vi "Initialize DO.vi"(0 "DAQ":refnum<class "DAQ.lvclass">, 5 "DAQNode Dict":T1, 7 "DO Channels":T2[](array[typedef]), 11 "error in":errorcluster, 14 "Simulate":bool) -> (4 "DAQ out":refnum<class "DAQ.lvclass">, 6 "DAQNode Dict out":T1, 15 "error out":errorcluster)   [LabVIEW 2017, in "DAQ.lvclass"]
doc: "Developed by Kevin Thompson\nkevin@thompsonengineering.net\n\nCopyright 2015\nThompson Engineering, LLC"
uses:
  DAQ.lvclass
  DataTypes/TD DO Channel--cluster.ctl
  <vilib>/TELLC/Dynamic CVT API/TD Dynamic CVT DVR--ref.ctl
  DAQ.lvclass/DAQ.ctl
  Accessors/Set DO IONames.vi
  Accessors/Set DO SchemNames.vi
  <vilib>/DAQmx/create/channels.llb/DAQmx Create Channel (DO-Digital Output).vi
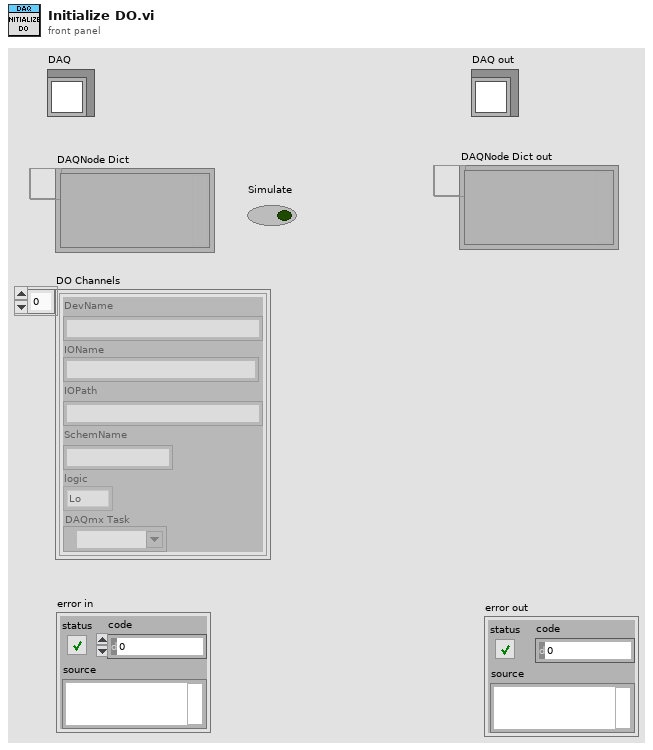
[diagram p1: front panel]
types:
  T1 = typedef "TD Dynamic CVT DVR--ref.ctl" = refnum<data-value>
  T2 = typedef "DAQ.lvclass/TD DO Channel--cluster.ctl" = cluster{"DevName":string, "IOName":string, "IOPath":string, "SchemName":string, "logic":enum16{"Lo", "Hi"}, "DAQmx Task":refnum<k21>}
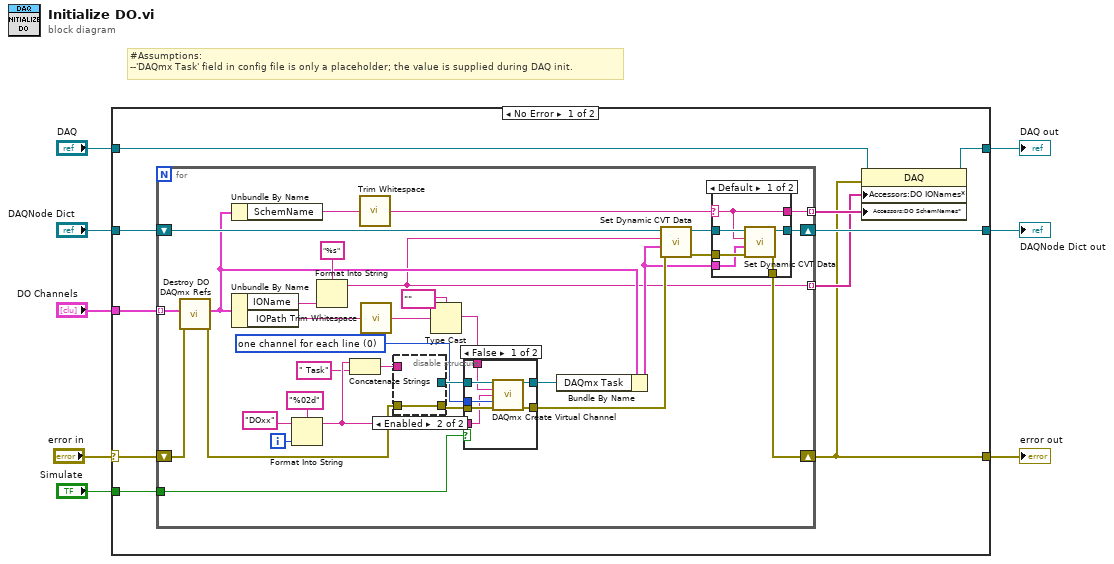
[diagram p0: block diagram]
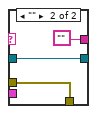
[diagram p2: hidden frame]
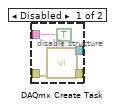
[diagram p3: hidden frame]
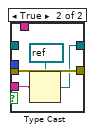
[diagram p4: hidden frame]
diagram:
  # "#Assumptions:\n--'DAQmx Task' field in config file is only a placeholder; the value is supplied during DAQ init."
  n1 = case shown="No Error" "error in" {
    selector: "error in" -> [w17 w79]
    tunnel: "DO Channels" -> [w16 _]
    tunnel: "DAQNode Dict" -> [w18 w78]
    tunnel: [w12 w79] -> w6
    tunnel: [w15 w78] -> w5
    tunnel: "Simulate" -> [w9 _]
    tunnel: "DAQ" -> [w11 w77]
    tunnel: [w10 w77] -> w1
    frame No Error {
      n2 = for {
        tunnel: w16 -> [w36] mode=indexing
        shift-right: [w26] -> w12
        shift-left: w17 -> [w35]
        shift-right: [w28] -> w15
        shift-left: w18 -> [w44]
        tunnel: [w21] -> w14 mode=indexing
        tunnel: [w20] -> w13 mode=indexing
        tunnel: w9 -> [w19]
        i -> [w47]
        w42 = 0 items=["one channel for each line", "one channel for all lines"] ("line grouping")
        n3 = call "Destroy DO DAQmx Refs.vi"("error in (no error)"=w35, "DO"=w36) -> ("error out"=w34:errorcluster, "DO out"=w24:T2)  [unwired: 8 in]
        n4 = Unbundle By Name(w24) -> ("SchemName"=w23:string)
        n5 = Unbundle By Name(w24) -> ("IOName"=w33:string, "IOPath"=w49:string)
        n6 = Format Into String(format string="%02d", initial string="DOxx", w47) -> (resulting string=w39:string)  [unwired: 1 in, 1 out]
        n7 = Format Into String(format string="%s", w33) -> (resulting string=w20:string)  [unwired: 2 in, 1 out]
        n8 = Concatenate Strings(w39, " Task" ("string")) -> (w37:string)
        n9 = call <vilib>:"Trim Whitespace.vi"("string"=w23) -> ("trimmed string"=w22:string)  [unwired: 1 in]
        n10 = call <vilib>:"Trim Whitespace.vi"("string"=w49) -> ("trimmed string"=w48:string)  [unwired: 1 in]
        n11 = disable-structure shown="Enabled" {
          disable-tunnel: [w64 _] -> w50
          disable-tunnel: [w63 w65] -> w45
          disable-tunnel: w37 -> [w62 _]
          disable-tunnel: w34 -> [w61 w65]
          frame Disabled {
            n12 = call <vilib>:"DAQmx Create Task.vi"("new task name"=w62, "auto cleanup"=TRUE, "error in"=w61) -> ("task out"=w64:refnum<k21>, "error out"=w63:errorcluster)  [unwired: 11 in]
          }
          frame Enabled {
          }
        }
        n13 = Type Cast(type=tag "" ("lines"), x=w48) -> (*(type *) &x=w40:tag)
        n14 = case shown="False" w19 {
          tunnel: w50 -> [w72 _]
          tunnel: w45 -> [w71 w76]
          tunnel: [w70 w73] -> w43
          tunnel: [w69 w76] -> w31
          tunnel: w42 -> [w68 _]
          tunnel: w40 -> [w67 _]
          tunnel: w39 -> [w66 w75]
          frame False {
            n15 = call-poly <vilib>:"DAQmx Create Virtual Channel.vi"("task in"=w72, "lines"=w67, "name to assign"=w66, "line grouping"=w68, "error in"=w71) -> ("task out"=w70:refnum<k21>, "error out"=w69:errorcluster)  [unwired: 9 in]
          }
          frame True {
            n16 = Type Cast(type=refnum<k21> refnum ("task out"), x=w75) -> (*(type *) &x=w73:refnum<k21>)
          }
        }
        n17 = Bundle By Name(cluster=w24, "DAQmx Task"=w43) -> (w25:T2)
        n18 = call <vilib>:"Set Dynamic CVT Data.vi"("error in (no error)"=w31, "value"=w25, "DataName"=w20, "dCVT DVR"=w44) -> ("error out"=w27:errorcluster, "dCVT DVR out"=w29:T1)  [unwired: 5 in, 1 out]
        n19 = case shown="Default" w22 {
          selector: w22 -> [w51 _]
          tunnel: w29 -> [w56 w59]
          tunnel: [w55 w59] -> w28
          tunnel: w27 -> [w54 w58]
          tunnel: [w53 w58] -> w26
          tunnel: w25 -> [w52 _]
          tunnel: [w51 ""] -> w21
          frame Default {
            n20 = call <vilib>:"Set Dynamic CVT Data.vi"("error in (no error)"=w54, "value"=w52, "DataName"=w51, "dCVT DVR"=w56) -> ("error out"=w53:errorcluster, "dCVT DVR out"=w55:T1)  [unwired: 5 in, 1 out]
          }
          frame "" {
          }
        }
      }
      n21 = property class="DAQ"(reference=w11, error in=w12, "Accessors:DO IONames*"=w13, "Accessors:DO SchemNames*"=w14) -> (reference out=w10:refnum<class "DAQ.lvclass">)  [unwired: 1 out]
    }
    frame Error {
    }
  }
  "error out" <- w6
  "DAQNode Dict out" <- w5
  "DAQ out" <- w1
